vi "CCP_display_image.vi"(7 "folder_name":string="image", 8 "error in":errorcluster, 11 "file_name":string="Shell_Volume.png") -> (0 "error out":errorcluster, 3 "status":bool, 4 "path":path)   [LabVIEW 2019]
panel:
  in  "command":string="rundll32 \"C:\\Program Files\\Windows Photo Viewer\\PhotoViewer.dll\",ImageView_Fullscreen"
  # "Sub-VI to display an image file using Windows Photo Viewer."
  # "Relative to this VI."
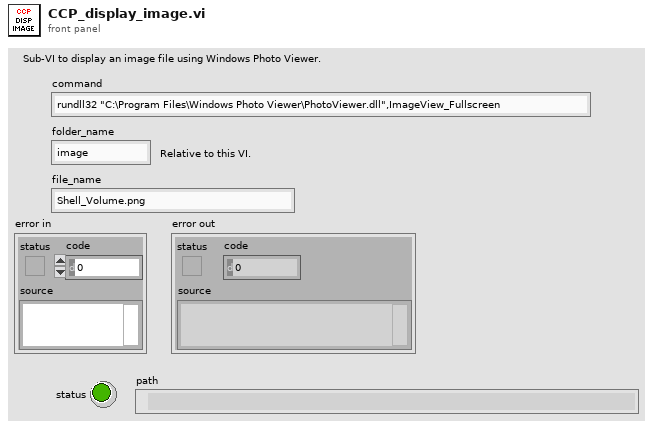
[diagram p1: front panel]
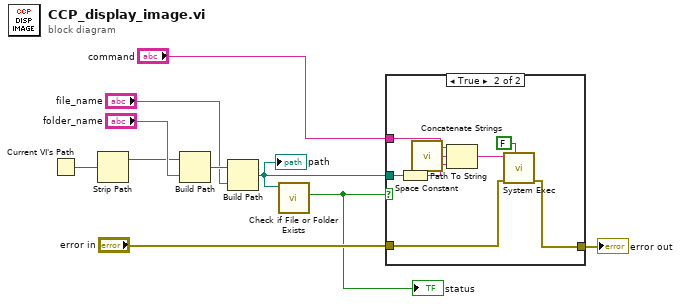
[diagram p0: block diagram]
diagram:
  n1 = Current VI's Path() -> (path=w1:path)
  n2 = Strip Path(path=w1) -> (stripped path=w2:path)  [unwired: 1 out]
  n3 = Build Path(base path=w2, name or relative path="folder_name") -> (appended path=w5:path)
  n4 = Build Path(base path=w5, name or relative path="file_name") -> (appended path=w7:path)
  "path" <- w7
  n5 = call <vilib>:"Check if File or Folder Exists.vi"("path"=w7) -> ("file or folder exists?"=w8:bool)  [unwired: 8 in, 2 out]
  "status" <- w8
  n6 = case shown="True" w8 {
    tunnel: "error in" -> [w11 w14]
    tunnel: [w11 w13] -> w9
    tunnel: w7 -> [_ w19]
    tunnel: "command" -> [_ w16]
    frame False {
    }
    frame True {
      n7 = Path To String(path=w19) -> (string=w18:string)
      n8 = call <vilib>:"Space Constant.vi"() -> ("String"=w17:string)
      n9 = Concatenate Strings(w16, w17, w18) -> (w15:string)
      n10 = call <vilib>:"System Exec.vi"("wait until completion? (T)"=FALSE, "error in (no error)"=w14, "command line"=w15) -> ("error out"=w13:errorcluster)  [unwired: 5 in, 3 out]
    }
  }
  "error out" <- w9
